vi "Channel ID to Wave ID.vi"(10 "Ch N":T1, 11 "Channel ID":i16) -> (3 "Wave ID":i16)   [LabVIEW 2015]
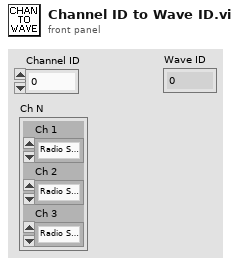
[diagram p1: front panel]
types:
  T1 = cluster{"Ch 1":enum32{"Radio Selection 1", "Radio Selection 2", "Radio Selection 3"}, "Ch 2":enum32{"Radio Selection 1", "Radio Selection 2", "Radio Selection 3"}, "Ch 3":enum32{"Radio Selection 1", "Radio Selection 2", "Radio Selection 3"}}
  T2 = enum32{"Radio Selection 1", "Radio Selection 2", "Radio Selection 3"}
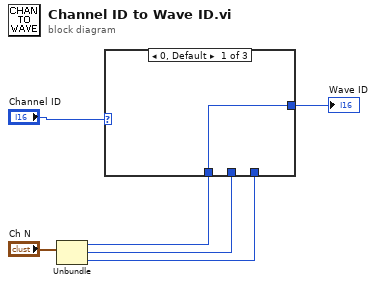
[diagram p0: block diagram]
diagram:
  n1 = Unbundle("Ch N") -> ("Ch 1"=w3:T2, "Ch 2"=w2:T2, "Ch 3"=w1:T2)
  n2 = case shown="0, Default" "Channel ID" {
    tunnel: [w7 w8 w9] -> w5
    tunnel: w3 -> [w7 _ _]
    tunnel: w2 -> [_ w8 _]
    tunnel: w1 -> [_ _ w9]
    frame 0, Default {
    }
    frame 1 {
    }
    frame 2 {
    }
  }
  "Wave ID" <- w5
